vi "Scan Status View.vi"(10 "UserEvents in":refnum<class "UserEvents.lvclass">) -> ()   [LabVIEW 2015, in "FAMT Views.lvlib"]
uses:
  FAMT Views.lvlib
  UserEvents/UserEvents.lvclass
  UserEvents/UserEvents.lvclass/UserEvents.ctl
  Typedefs/State Types.ctl
  Typedefs/FAMT Typedefs.lvlib
panel:
  out "Waveform Step":u16
  out "State":string
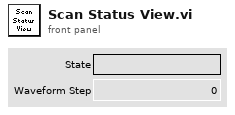
[diagram p1: front panel]
types:
  T1 = typedef "FAMT Typedefs.lvlib/Publish Data Events.ctl" = cluster{"State":refnum<user-event>, "ErrorCode":refnum<user-event>, "FC1 ILC Outputs":refnum<user-event>, "LogPath":refnum<user-event>, "FC1 ILC Inputs":refnum<user-event>, "Scan Progress":refnum<user-event>, "FC2 ILC Outputs":refnum<user-event>, "FC2 ILC Inputs":refnum<user-event>}
  T2 = cluster{"Event Registration Refnum":refnum<event-registration>, "Event Registration Refnum":refnum<event-registration>}
  T3 = typedef "FAMT Typedefs.lvlib/State Types.ctl" = enum16{"Offline State", "Fault State", "Standby State", "Disabled State", "Enabled State", "Wait For User Input State", "Perform Scan State"}
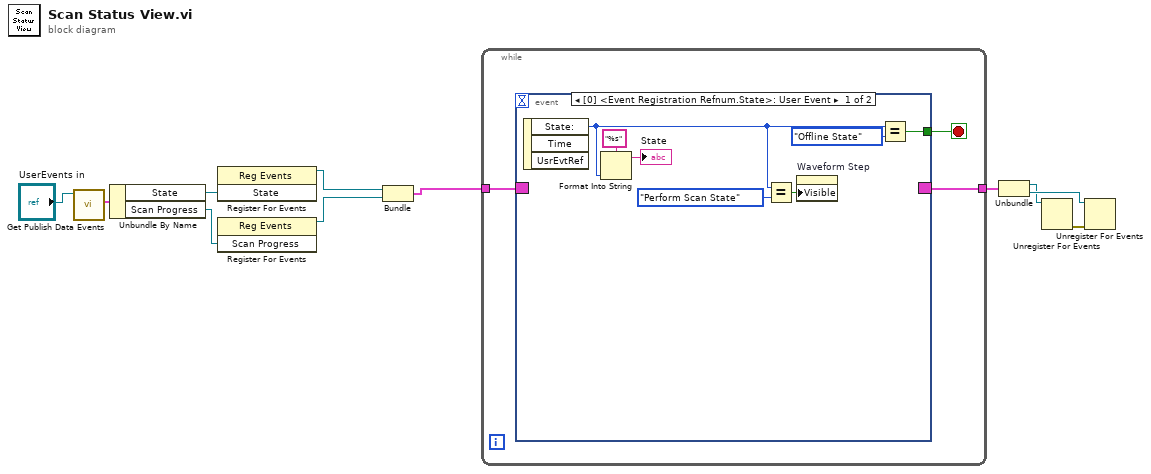
[diagram p0: block diagram]
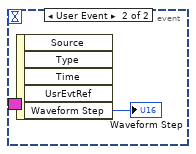
[diagram p2: hidden frame]
diagram:
  n1 = call "Get Publish Data Events.vi"("UserEvents in"="UserEvents in") -> ("Publish Data Events"=w10:T1)  [unwired: 9 in, 1 out]
  n2 = Unbundle By Name(w10) -> ("State"=w9:refnum<user-event>, "Scan Progress"=w11:refnum<user-event>)
  n3 = register-events(w9) -> (reference out=w4:refnum<event-registration>)  [unwired: 2 in, 1 out]
  n4 = register-events(w11) -> (reference out=w5:refnum<event-registration>)  [unwired: 2 in, 1 out]
  n5 = Bundle("Event Registration Refnum"=w4, "Event Registration Refnum"=w5) -> (w3:T2)  [unwired: 1 in]
  n6 = while {
    tunnel: w3 -> [w14]
    tunnel: [w13] -> w2
    stop <- w12 stop-if-true
    n7 = event shown="[0] <Event Registration Refnum.State>: User Event" {
      selector: w14 -> [_ _]
      dyn-events: [_ _] -> w13
      timeout: _ -> [_ _]
      tunnel: [w20 _] -> w12
      event User Event {
        n8 = event-data() -> ("State:"=w16:T3)  [unwired: 1 in, 2 out]
        n9 = Format Into String(format string="%s", w16) -> (resulting string=→"State":string)  [unwired: 2 in, 1 out]
        n10 = Equal?(x=w16, y=State_Types."Perform Scan State") -> (x = y?=w17:bool)
        n11 = property on="Waveform Step" class="DigNum (strict)"("Visible"=w17) -> ()  [unwired: 2 in, 2 out]
        n12 = Equal?(x=w16, y=State_Types."Offline State") -> (x = y?=w20:bool)
      }
      event User Event {
        n13 = event-data() -> ("Waveform Step"=→"Waveform Step":u16)  [unwired: 1 in, 4 out]
      }
    }
  }
  n14 = Unbundle(w2) -> ("Event Registration Refnum"=w1:refnum<event-registration>, "Event Registration Refnum"=w6:refnum<event-registration>)
  n15 = Unregister For Events(event registration refnum=w1) -> (error out=w7:errorcluster)  [unwired: 1 in]
  n16 = Unregister For Events(event registration refnum=w6, error in=w7) -> ()  [unwired: 1 out]
